vi "Finalize.vi"(8 "error in":errorcluster, 11 "logging execution unit in":refnum<class "Logging Execution Unit.lvclass">) -> (0 "error out":errorcluster, 3 "logging execution unit out":refnum<class "Logging Execution Unit.lvclass">)   [LabVIEW 2020, in "Ballard MIL-STD-1553 Engine.lvlib" / "Implementation.lvlib" / "Logging Execution Unit.lvclass"]
uses:
  Logging Execution Unit.lvclass
  C:/Git/niveristand-ballard-milStd1553-custom-device/Source/Custom Device Support/Engine/Implementation/Execution Unit/Execution Unit.lvclass
  Execution Unit/Execution Unit.lvclass/Execution Unit.ctl
  Execution Unit/Execution Unit.lvclass
  <instrlib>/BTICardLib/BTICardLV.lvlib
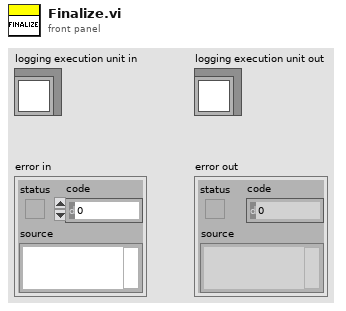
[diagram p1: front panel]
types:
  T1 = typedef "Ballard MIL-STD-1553 Engine.lvlib/Custom Device.lvlib/Hardware Handles.ctl" = cluster{"core handle":u64, "core reader handle":u64, "channel handles":u64[]}
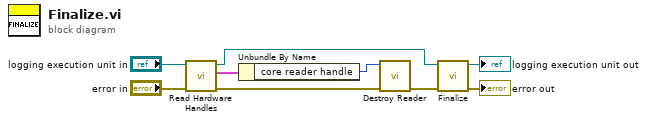
[diagram p0: block diagram]
diagram:
  n1 = call "Read Hardware Handles.vi"("error in"="error in", "Execution Unit in"="logging execution unit in") -> ("error out"=w2:errorcluster, "hardware handles"=w4:T1, "Execution Unit out"=w1:refnum<class "Logging Execution Unit.lvclass">)  [unwired: 7 in]
  n2 = Unbundle By Name(w4) -> ("core reader handle"=w3:u64)
  n3 = call <instrlib>:"Destroy Reader.vi"("error in (no error)"=w2, "reader handle in"=w3) -> ("error out"=w7:errorcluster)  [unwired: 9 in]
  n4 = call-parent "Finalize.vi"("error in (no error)"=w7, "Execution Unit Implementation in"=w1) -> ("error out"=→"error out":errorcluster, "Execution Unit Implementation out"=→"logging execution unit out":refnum<class "Logging Execution Unit.lvclass">)  [unwired: 8 in]
